vi "Frame Set w.vi"(8 "error in (no error)":errorcluster, 10 "<w> Data":T1, 11 "IDE simple in":refnum<class "LF2R IDE.lvclass">) -> (0 "error out":errorcluster, 3 "IDE simple out":refnum<class "LF2R IDE.lvclass">)   [LabVIEW 2018, in "LF2R IDE.lvlib" / "LF2R IDE.lvclass"]
uses:
  LF2R IDE.lvclass
  Frame Analizer/frame w data.ctl
  LF2R IDE.lvclass/LF2R IDE.ctl
  Frame Analizer/Data Parser.lvclass
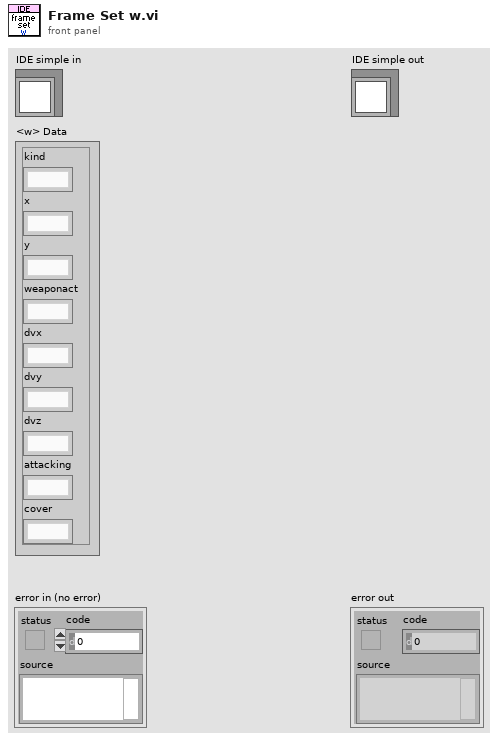
[diagram p1: front panel]
types:
  T1 = typedef "Data Parser.lvclass/frame w data.ctl" = cluster{"kind":string, "x":string, "y":string, "weaponact":string, "dvx":string, "dvy":string, "dvz":string, "attacking":string, "cover":string}
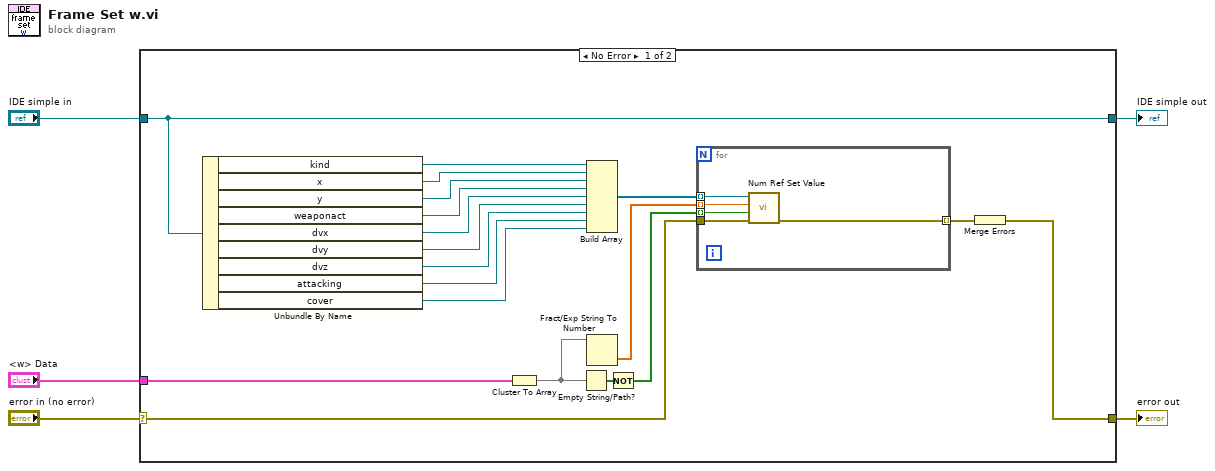
[diagram p0: block diagram]
diagram:
  n1 = case shown="No Error" "error in (no error)" {
    selector: "error in (no error)" -> [w23 w31]
    tunnel: [w19 w31] -> w4
    tunnel: [w15 w30] -> w2
    tunnel: "IDE simple in" -> [w15 w30]
    tunnel: "<w> Data" -> [w18 _]
    frame No Error {
      n2 = Unbundle By Name(w15) -> ("kind"=w14:refnum<vi>, "x"=w13:refnum<vi>, "y"=w12:refnum<vi>, "weaponact"=w11:refnum<vi>, "dvx"=w10:refnum<vi>, "dvy"=w9:refnum<vi>, "dvz"=w8:refnum<vi>, "attacking"=w7:refnum<vi>, "cover"=w6:refnum<vi>)
      n3 = Cluster To Array(cluster=w18) -> (array=w17:string[])
      n4 = Empty String/Path?(string/path=w17) -> (empty?=w24:bool[])
      n5 = Build Array(w14, w13, w12, w11, w10, w9, w8, w7, w6) -> (w16:refnum<vi>[])
      n6 = Fract/Exp String To Number(string=w17) -> (number=w21:dbl[])  [unwired: 3 in, 1 out]
      n7 = Not(x=w24) -> (.not. x?=w22:bool[])
      n8 = for {
        tunnel: w23 -> [w29]
        tunnel: w16 -> [w25] mode=indexing
        tunnel: w22 -> [w26] mode=indexing
        tunnel: w21 -> [w28] mode=indexing
        tunnel: [w27] -> w20 mode=indexing
        n9 = call "Num Ref Set Value.vi"("error in"=w29, "Valid"=w26, "Value"=w28, "Num Ref"=w25) -> ("error out"=w27:errorcluster)  [unwired: 7 in]
      }
      n10 = Merge Errors(w20) -> (w19:errorcluster)
    }
    frame Error {
    }
  }
  "error out" <- w4
  "IDE simple out" <- w2
